vi "Read.vi"(11 "EventsValue in":refnum<class "EventsValue.lvclass">) -> (2 "Events":T1[](array[typedef]))   [LabVIEW 2020, in "Volatus.lvlib" / "EventsValue.lvclass"]
uses:
  EventsValue.lvclass
  EventsValue.lvclass/EventsValue.ctl
  Event Level.ctl
  Volatus.lvlib
  Event.ctl
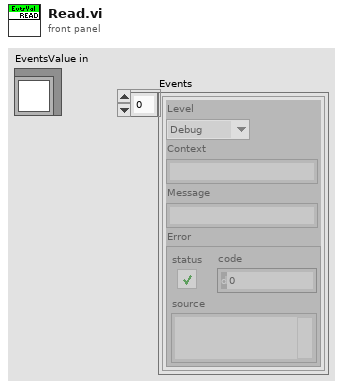
[diagram p1: front panel]
types:
  T1 = typedef "Volatus.lvlib/Event.ctl" = cluster{"Level":T2, "Context":string, "Message":string, "Error":errorcluster}
  T2 = typedef "Volatus.lvlib/Event Level.ctl" = enum16{"Debug", "Info", "Warning", "Error"}
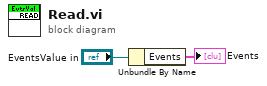
[diagram p0: block diagram]
diagram:
  n1 = Unbundle By Name("EventsValue in") -> ("Events"=→"Events":T1[])
